vi "Lock-In Ignore if not initialized.vi"(9 "Command in":T1=enum."Ignore", 11 "Initialized?":bool) -> (1 "Command out":T1=enum."Ignore")   [LabVIEW 2018, in "Lock-in module.lvlib"]
doc: "Returns enum with command to ignore message, if module is not initialized. In that case, only \"initialize\" command will be accepted."
uses:
  Lock-in module.lvlib
  ctl/MFLI_command enum.ctl
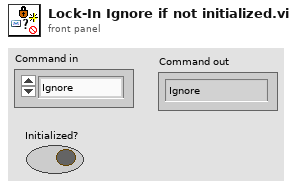
[diagram p1: front panel]
types:
  T1 = typedef "Lock-in module.lvlib/MFLI_command enum.ctl" = enum16{"Initialize", "Update", "Set parameters", "Set module", "Set individual parameters", "Get point", "Get array", "Disconnect", "End", "Ignore"}
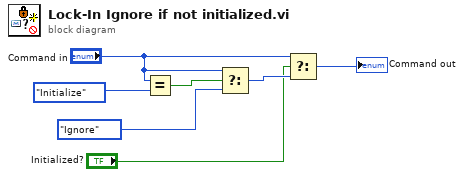
[diagram p0: block diagram]
diagram:
  n1 = Equal?(x="Command in", y=MFLI_command_enum."Initialize" ("Command in")) -> (x = y?=w6:bool)
  n2 = Select(t="Command in", s=w6, f=MFLI_command_enum."Ignore" ("Command in")) -> (s? t:f=w7:T1)
  n3 = Select(t="Command in", s="Initialized?", f=w7) -> (s? t:f=→"Command out":T1)
